vi "FormulaDeHeron.vi"(7 "c":dbl, 8 "b":dbl, 9 "a":dbl) -> (3 "Area Triangulo":dbl)   [LabVIEW 2018]
panel:
  # "Dimenciones Triangulo"
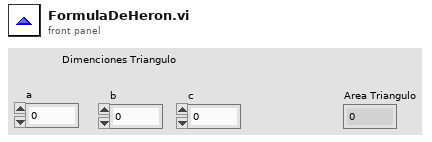
[diagram p1: front panel]
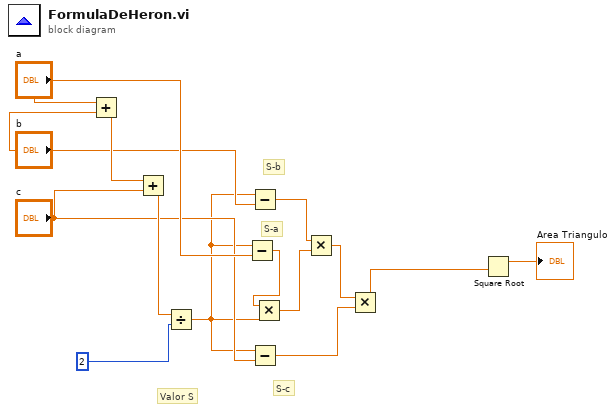
[diagram p0: block diagram]
diagram:
  # "S-c"
  # "S-b"
  # "S-a"
  # "Valor S"
  n1 = Add(x="a", y="b") -> (x+y=w13:dbl)
  n2 = Add(x=w13, y="c") -> (x+y=w12:dbl)
  n3 = Divide(x=w12, y=2) -> (x/y=w4:dbl)
  n4 = Subtract(x=w4, y="a") -> (x-y=w9:dbl)
  n5 = Subtract(x=w4, y="b") -> (x-y=w6:dbl)
  n6 = Subtract(x=w4, y="c") -> (x-y=w3:dbl)
  n7 = Multiply(x=w9, y=w4) -> (x*y=w7:dbl)
  n8 = Multiply(x=w6, y=w7) -> (x*y=w2:dbl)
  n9 = Multiply(x=w2, y=w3) -> (x*y=w1:dbl)
  n10 = Square Root(x=w1) -> (sqrt(x)=→"Area Triangulo":dbl)
